vi "Cluster Experiement.vi"() -> ()   [LabVIEW 2014]
panel:
  out "Small Cluster":cluster{"Boolean 1":bool, "Slide Value":dbl}
  out "Modified Cluster":T1 {"Slide" scale=0.0..10.0}
  in  "Cluster":T1 {"Slide" scale=0.0..10.0}
  out "Boolean 2":bool
  out "Numeric":dbl
  in  "stop":bool
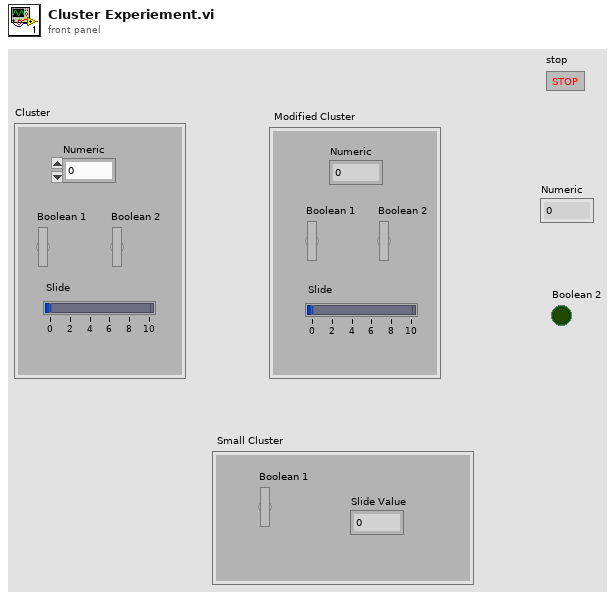
[diagram p1: front panel]
types:
  T1 = cluster{"Numeric":dbl, "Boolean 1":bool, "Boolean 2":bool, "Slide":dbl}
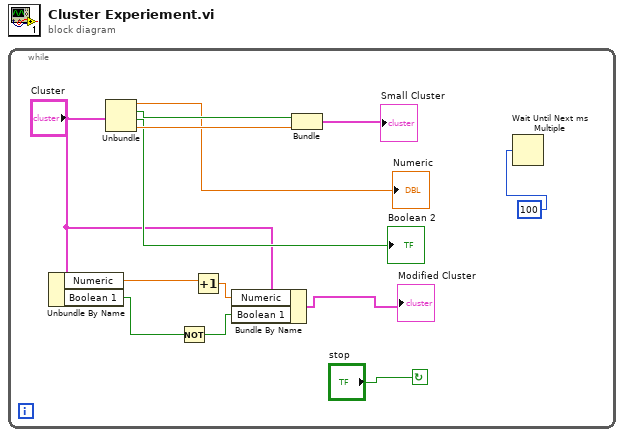
[diagram p0: block diagram]
diagram:
  n1 = while {
    stop <- "stop" continue-if-true
    n2 = Unbundle By Name("Cluster") -> ("Numeric"=w8:dbl, "Boolean 1"=w7:bool)
    n3 = Unbundle("Cluster") -> ("Numeric"=→"Numeric":dbl, "Boolean 1"=w12:bool, "Boolean 2"=→"Boolean 2":bool, "Slide"=w11:dbl)
    n4 = Not(x=w7) -> (.not. x?=w3:bool)
    n5 = Increment(x=w8) -> (x+1=w4:dbl)
    n6 = Bundle By Name(cluster="Cluster", "Numeric"=w4, "Boolean 1"=w3) -> (→"Modified Cluster":T1)
    n7 = Bundle("Boolean 1"=w12, "Slide"=w11) -> (→"Small Cluster":cluster{"Boolean 1":bool, "Slide":dbl})  [unwired: 1 in]
    n8 = Wait Until Next ms Multiple(millisecond multiple=100) -> ()  [unwired: 1 out]
  }
